vi "FTW-Connector-LaunchActor.vi"(0 "FTW Actor Connector":refnum<class "FTW-Actor-Connector.lvclass">, 5 "Actor Instance Configuration":string, 11 "error in":errorcluster) -> (4 "FTW Actor Connector out":refnum<class "FTW-Actor-Connector.lvclass">, 15 "error out":errorcluster)   [LabVIEW 2013, in "FTW-Actor-Connector.lvclass"]
doc: "Spawns a new Actor Instance given an Actor Instance Configuration.\n\nThis method is dynamic dispatch, enabling any launch topology desired by Connector subclasses, including statically linking the Instance Process (it's dynamically linked by default to decouple Connector from Instance), or creating a new Connector Pane for the Instance Process."
uses:
  FTW-Actor-Connector.lvclass
  lib/jansson/FTWLib-JSON-LibraryFilepath.vi
  json/lib/FTW-JSON-Core-LibraryError.vi
  error/FTW-ERR-ThrowGenericError.vi
  error/FTW-ERR-ThrowError.vi
  reflection/FTW-Reflection-Type.vi
  error/FTW-ERR-CallChain.vi
  string/FTW-STR-ReplaceWhitespace.vi
  json/lib/FTW-JSON-Core-GetFlattenedValue.vi
  json/FTW-JSON-Deserialize/FTW-JSON-Deserialize.xnode
panel:
  # "Inputs"
  # "Outputs"
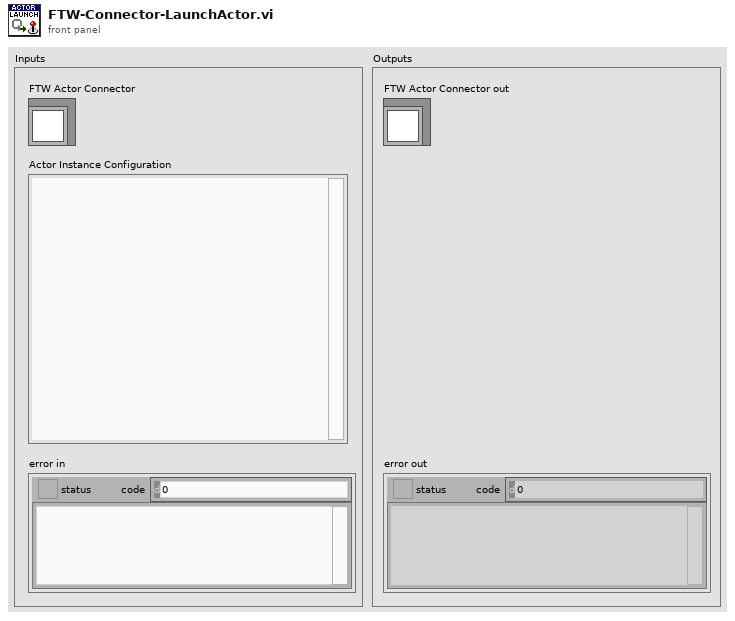
[diagram p1: front panel]
types:
  T1 = cluster{"DebugShowPanel":bool, "ActorInstanceVIFilepath":path, "ActorInstanceVIName":string}
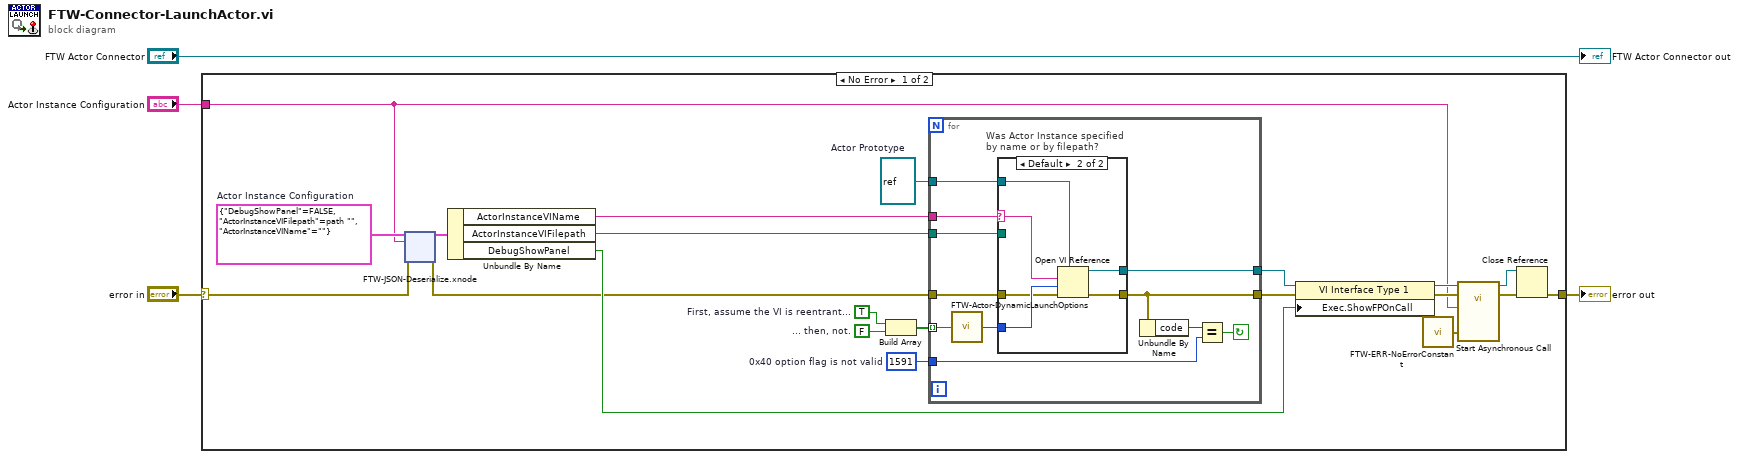
[diagram p0: block diagram]
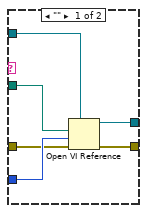
[diagram p2: hidden frame]
diagram:
  n1 = case shown="No Error" "error in" {
    selector: "error in" -> [w14 w83]
    tunnel: [w24 w83] -> w4
    tunnel: "Actor Instance Configuration" -> [w13 _]
    frame No Error {
      w7 = 1591  # 0x40 option flag is not valid
      w10 = FALSE  # ... then, not.
      w11 = TRUE  # First, assume the VI is reentrant...
      w20 = T1 {"DebugShowPanel"=FALSE, "ActorInstanceVIFilepath"=path "", "ActorInstanceVIName"=""}  # Actor Instance Configuration
      w25 = refnum<vi> refnum  # Actor Prototype
      n2 = xnode "FTW-JSON-Deserialize.xnode"("Type and Defaults"=w20, "JSON String"=w13, "error in"=w14) -> ("Values"=w21:T1, "error out"=w8:errorcluster)
      n3 = Unbundle By Name(w21) -> ("ActorInstanceVIName"=w5:string, "ActorInstanceVIFilepath"=w6:path, "DebugShowPanel"=w23:bool)
      n4 = Build Array(w11, w10) -> (w9:bool[])
      n5 = for {
        tunnel: w25 -> [w36]
        tunnel: [w34] -> w22
        tunnel: [w30] -> w12
        tunnel: w9 -> [w33] mode=indexing
        tunnel: w8 -> [w32]
        tunnel: w7 -> [w31]
        tunnel: w6 -> [w27]
        tunnel: w5 -> [w26]
        stop <- w28 continue-if-true
        n6 = call "FTW-Actor-DynamicLaunchOptions.vi"("Reentrant?"=w33) -> ("Open VI Ref Options"=w35:i32)
        n7 = case "Was Actor Instance specified\nby name or by filepath?" shown="Default" w26 {
          selector: w26 -> [_ w43]
          tunnel: w36 -> [w42 w48]
          tunnel: w35 -> [w41 w47]
          tunnel: [w40 w46] -> w34
          tunnel: w32 -> [w39 w45]
          tunnel: [w38 w44] -> w30
          tunnel: w27 -> [w37 _]
          frame "" {
            n8 = Open VI Reference(type specifier VI Refnum (for type only)=w42, vi path=w37, options=w41, error in (no error)=w39) -> (vi reference=w40:refnum<vi>, error out=w38:errorcluster)  [unwired: 2 in]
          }
          frame Default {
            n9 = Open VI Reference(type specifier VI Refnum (for type only)=w48, vi path=w43, options=w47, error in (no error)=w45) -> (vi reference=w46:refnum<vi>, error out=w44:errorcluster)  [unwired: 2 in]
          }
        }
        n10 = Unbundle By Name(w30) -> ("code"=w29:i32)
        n11 = Equal?(x=w29, y=w31) -> (x = y?=w28:bool)
      }
      n12 = property class="VI Interface Type 1"(reference=w22, error in=w12, "Exec.ShowFPOnCall"=w23) -> (reference out=w19:refnum<vi>, error out=w18:errorcluster)
      n13 = call "FTW-ERR-NoErrorConstant.vi"() -> ("no error"=w17:errorcluster)
      n14 = call-by-ref "Start Asynchronous Call"(reference=w19, error in=w18, "FTW Actor Instance Configuration"=w13, "ErrorIn"=w17) -> (reference out=w15:refnum<vi>, error out=w16:errorcluster)  [unwired: 13 in, 1 out]
      n15 = Close Reference(reference=w15, error in (no error)=w16) -> (error out=w24:errorcluster)
    }
    frame Error {
    }
  }
  "error out" <- w4
  "FTW Actor Connector out" <- "FTW Actor Connector"
